vi "Get Label Settings for RT.vi"(8 "error in":errorcluster, 11 "label ref in":T1 format="%.0x") -> (0 "error out":errorcluster, 2 "label settings for RT":T2 {"Label Timestamp Channel Data Reference" format="%.0x"; "Word Initial Raw Value" format="%032.0f"; "Label Disable/Trigger Channel Reference" format="%.0x"; "parameter driver data"."Tx parameter refs" format="%.0x"; "parameter driver data"."Rx block data refs"."Data Reference" format="%.0x"; "SDI" format="%02b"; "label" format="%.0o"}, 3 "label ref out":T1 format="%.0x")   [LabVIEW 2020]
uses:
  <vilib>/NI VeriStand/Custom Device API/Custom Device API.lvlib
  <vilib>/NI VeriStand/Custom Device API/Get Item Property (U32).vi
  Scripting/Constants.vi
  Scripting/Ballard ARINC 429 Scripting.lvlib
  Transfer Type.ctl
  <vilib>/NI VeriStand/Custom Device API/Custom Device Item Ref.ctl
  <vilib>/NI VeriStand/Custom Device API/Data Reference.ctl
  <vilib>/NI VeriStand/Custom Device API/Block Data Reference.ctl
  Encoding and Decoding/Encoding.ctl
  Encoding and Decoding/Encoding and Decoding.lvlib
  RT Parameters.ctl
  Label.ctl
  RT Label Settings.ctl
  Parameter Definition.ctl
  <vilib>/NI VeriStand/Custom Device API/Get Item Property (U16).vi
  <vilib>/NI VeriStand/Custom Device API/Get Item Property (Boolean).vi
  <vilib>/NI VeriStand/Custom Device API/Get Item Property (String).vi
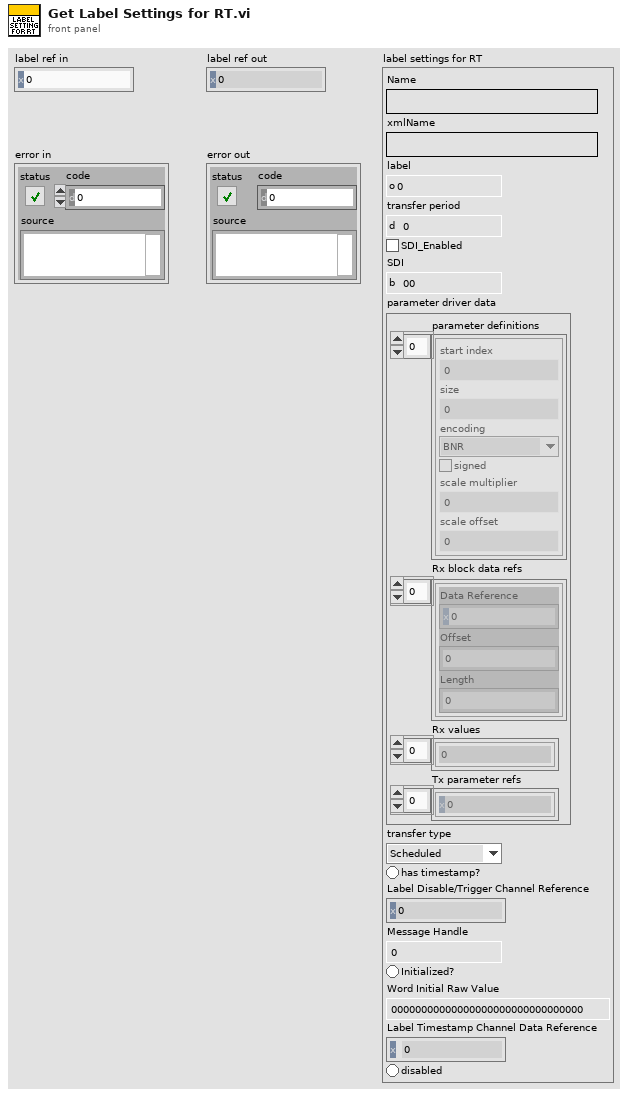
[diagram p1: front panel]
types:
  T1 = typedef "Custom Device API.lvlib/Custom Device Item Ref.ctl" = u64
  T2 = typedef "RT Label Settings.ctl" = cluster{"Name":string, "xmlName":string, "label":T3, "transfer period":u32, "SDI_Enabled":bool, "SDI":u8, "parameter driver data":T4, "transfer type":T9, "has timestamp?":bool, "Label Disable/Trigger Channel Reference":T1, "Message Handle":u64, "Initialized?":bool, "Word Initial Raw Value":u32, "Label Timestamp Channel Data Reference":T8, "disabled":bool}
  T3 = typedef "Label.ctl" = u8
  T4 = typedef "RT Parameters.ctl" = cluster{"parameter definitions":T5[], "Rx block data refs":T7[], "Rx values":dbl[], "Tx parameter refs":T1[]}
  T5 = typedef "Parameter Definition.ctl" = cluster{"start index":i32, "size":i32, "encoding":T6, "signed":bool, "scale multiplier":dbl, "scale offset":dbl}
  T6 = typedef "Encoding and Decoding.lvlib/Encoding.ctl" = enum16{"BNR", "BCD", "Discrete"}
  T7 = typedef "Custom Device API.lvlib/Block Data Reference.ctl" = cluster{"Data Reference":T8, "Offset":u64, "Length":u64}
  T8 = typedef "Custom Device API.lvlib/Data Reference.ctl" = i32
  T9 = typedef "Transfer Type.ctl" = enum16{"Scheduled", "Acyclic", "Block", "Strobe"}
  T10 = typedef "Custom Device API.lvlib/Custom Device Item Info.ctl" = cluster{"Name":string, "Is Channel":bool, "GUID":string, "Is Waveform":bool}
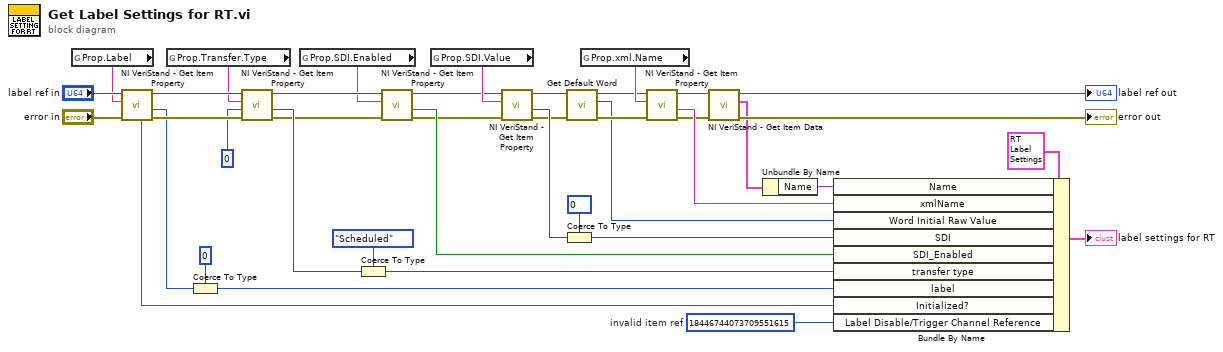
[diagram p0: block diagram]
diagram:
  w8 = T1 18446744073709551615  # invalid item ref
  n1 = global read "Constants.vi" "Prop.Label"() -> (w13:string)
  n2 = call-poly <vilib>:"NI VeriStand - Get Item Property.vi"("error in (no error)"="error in", "Property Name"=w13, "Item Ref in"="label ref in") -> ("error out"=w21:errorcluster, "Value"=w2:u32, "Item Ref out"=w20:T1, "Found?"=w1:bool)  [unwired: 5 in]
  n3 = global read "Constants.vi" "Prop.Transfer.Type"() -> (w19:string)
  n4 = Coerce To Type(0:w2, 1:T3 0 ("label")) -> (2:w36:T3)
  n5 = call-poly <vilib>:"NI VeriStand - Get Item Property.vi"("error in (no error)"=w21, "Default Value"=u16 0, "Property Name"=w19, "Item Ref in"=w20) -> ("error out"=w22:errorcluster, "Value"=w33:u16, "Item Ref out"=w23:T1)  [unwired: 4 in, 1 out]
  n6 = global read "Constants.vi" "Prop.SDI.Enabled"() -> (w16:string)
  n7 = Coerce To Type(0:w33, 1:Transfer_Type."Scheduled" ("transfer type")) -> (2:w34:T9)
  n8 = call-poly <vilib>:"NI VeriStand - Get Item Property.vi"("error in (no error)"=w22, "Property Name"=w16, "Item Ref in"=w23) -> ("error out"=w12:errorcluster, "Value"=w31:bool, "Item Ref out"=w11:T1)  [unwired: 5 in, 1 out]
  n9 = global read "Constants.vi" "Prop.SDI.Value"() -> (w17:string)
  n10 = call-poly <vilib>:"NI VeriStand - Get Item Property.vi"("error in (no error)"=w12, "Property Name"=w17, "Item Ref in"=w11) -> ("error out"=w6:errorcluster, "Value"=w29:u32, "Item Ref out"=w7:T1)  [unwired: 5 in, 1 out]
  n11 = Coerce To Type(0:w29, 1:u8 0 ("SDI")) -> (2:w30:u8)
  n12 = call "Get Default Word.vi"("error in"=w6, "Item Ref in"=w7) -> ("error out"=w4:errorcluster, "default word"=w3:u32, "Item Ref out"=w5:T1)  [unwired: 7 in]
  n13 = global read "Constants.vi" "Prop.xml.Name"() -> (w18:string)
  n14 = call-poly <vilib>:"NI VeriStand - Get Item Property.vi"("error in (no error)"=w4, "Property Name"=w18, "Item Ref in"=w5) -> ("error out"=w25:errorcluster, "Value"=w37:string, "Item Ref out"=w24:T1)  [unwired: 5 in, 1 out]
  n15 = call <vilib>:"NI VeriStand - Get Item Data.vi"("error in (no error)"=w25, "Item Ref in"=w24) -> ("error out"=→"error out":errorcluster, "Item Info"=w9:T10, "Item Ref out"=→"label ref out":T1)  [unwired: 6 in, 1 out]
  n16 = Unbundle By Name(w9) -> ("Name"=w27:string)
  n17 = Bundle By Name(cluster=T2 {"Name"="", "xmlName"="", "label"=0, "transfer period"=0, "SDI_Enabled"=FALSE, "SDI"=0, "parameter driver data"={"parameter definitions"=[], "Rx block data refs"=[], "Rx values"=[], "Tx parameter refs"=[]}, "transfer type"=enum."Scheduled", "has timestamp?"=FALSE, "Label Disable/Trigger Channel Reference"=0, "Message Handle"=0, "Initialized?"=FALSE, "Word Initial Raw Value"=0, "Label Timestamp Channel Data Reference"=0, "disabled"=FALSE} ("label settings for RT"), "Name"=w27, "xmlName"=w37, "Word Initial Raw Value"=w3, "SDI"=w30, "SDI_Enabled"=w31, "transfer type"=w34, "label"=w36, "Initialized?"=w1, "Label Disable/Trigger Channel Reference"=w8) -> (→"label settings for RT":T2)
